vi "CM-Endpoints to Channels.vi"(0 "Path":path, 2 "IO Type":string, 7 "Requested Endpoints":string[](array[string]), 11 "error in (no error)":errorcluster) -> (4 "IO Channels":string[](array[string]), 15 "error out":errorcluster)   [LabVIEW 2020]
uses:
  <vilib>/Utility/config.llb/Read Key (String).vi
  <vilib>/Utility/config.llb/NI_LVConfig.lvlib
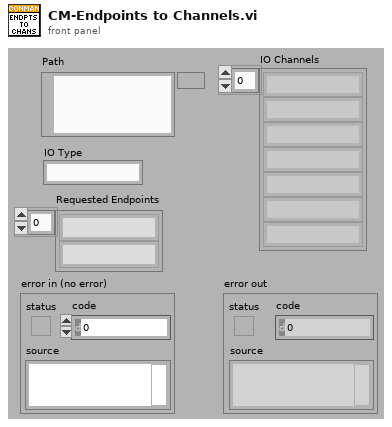
[diagram p1: front panel]
types:
  T1 = typedef "NI_LVConfig.lvlib/Config Data RefNum.ctl" = refnum<k1>
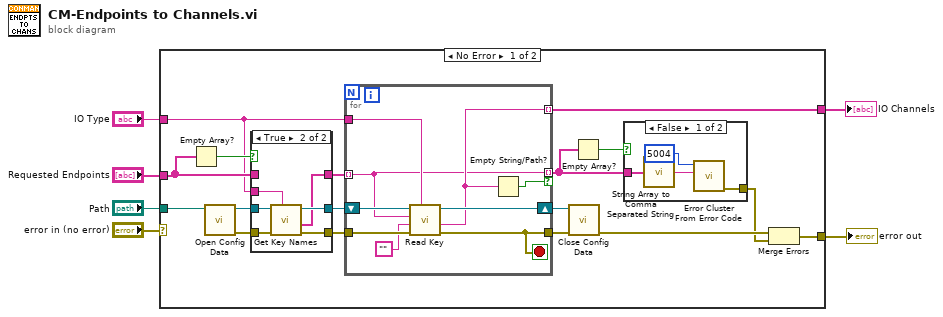
[diagram p0: block diagram]
diagram:
  n1 = case shown="No Error" "error in (no error)" {
    selector: "error in (no error)" -> [_ w46]
    tunnel: [w16 w46] -> w5
    tunnel: "Path" -> [w23 _]
    tunnel: "IO Type" -> [w7 _]
    tunnel: [w20 _] -> w2
    tunnel: "Requested Endpoints" -> [w11 _]
    frame No Error {
      n2 = Empty Array?(array=w11) -> (empty?=w13:bool)
      n3 = call <vilib>:"Open Config Data.vi"("configuration file path"=w23) -> ("error out"=w14:errorcluster, "refnum"=w10:T1)  [unwired: 8 in, 1 out]
      n4 = case shown="True" w13 {
        tunnel: w14 -> [w24 w32]
        tunnel: [w26 w28] -> w12
        tunnel: w11 -> [w26 _]
        tunnel: w10 -> [w25 w31]
        tunnel: [w25 w30] -> w9
        tunnel: [w24 w29] -> w8
        tunnel: w7 -> [_ w27]
        frame False {
        }
        frame True {
          n5 = call <vilib>:"Get Key Names.vi"("section"=w27, "error in (no error)"=w32, "refnum"=w31) -> ("error out"=w29:errorcluster, "key names"=w28:string[], "refnum out"=w30:T1)  [unwired: 5 in, 1 out]
        }
      }
      n6 = for {
        tunnel: w12 -> [w34] mode=indexing
        tunnel: w8 -> [w41]
        tunnel: [w37] -> w21
        tunnel: w7 -> [w38]
        shift-right: [w39] -> w22
        shift-left: w9 -> [w40]
        tunnel: [w35] -> w20 mode=indexing
        tunnel: [w34] -> w17 mode=indexing if=w33
        stop <- w37 stop-if-true
        n7 = call-poly <vilib>:"Read Key.vi"("section"=w38, "error in (no error)"=w41, "default value"="", "key"=w34, "refnum"=w40) -> ("error out"=w37:errorcluster, "value"=w35:string, "refnum out"=w39:T1)  [unwired: 3 in, 1 out]
        n8 = Empty String/Path?(string/path=w35) -> (empty?=w33:bool)
      }
      n9 = call <vilib>:"Close Config Data.vi"("error in (no error)"=w21, "refnum"=w22) -> ("error out"=w18:errorcluster)  [unwired: 8 in, 1 out]
      n10 = Empty Array?(array=w17) -> (empty?=w19:bool)
      n11 = case shown="False" w19 {
        tunnel: w17 -> [w45 _]
        tunnel: [w42 _] -> w15
        frame False {
          n12 = call "String Array to Comma Separated String.vi"("String Array"=w45) -> ("comma separated string"=w44:string)
          n13 = call <vilib>:"Error Cluster From Error Code.vi"("error message (\"\")"=w44, "error code (0)"=5004) -> ("error out"=w42:errorcluster)  [unwired: 7 in]
        }
        frame True {
        }
      }
      n14 = Merge Errors(w18, w15) -> (w16:errorcluster)
    }
    frame Error {
    }
  }
  "error out" <- w5
  "IO Channels" <- w2
